vi "something test.vi"(8 "error in (no error)":errorcluster, 11 "Dummy In":refnum<class "Dummy.lvclass">) -> (0 "error out":errorcluster, 3 "Dummy Out":refnum<class "Dummy.lvclass">)   [LabVIEW 2020, in "Dummy.lvclass"]
uses:
  Dummy.lvclass
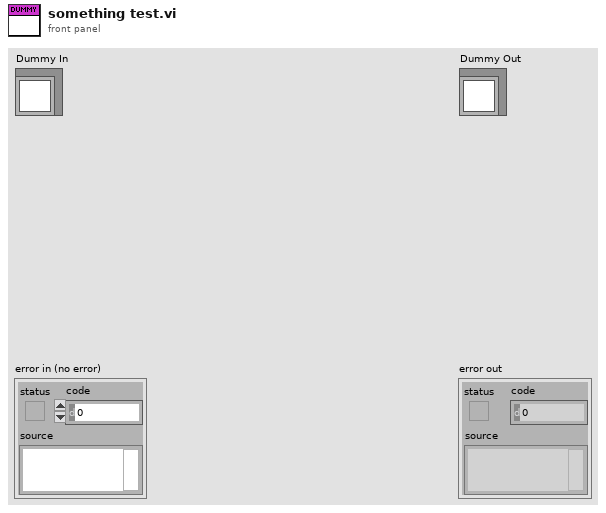
[diagram p1: front panel]
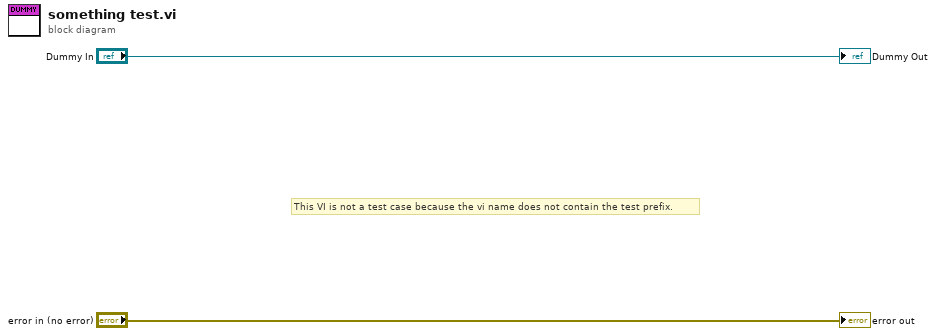
[diagram p0: block diagram]
diagram:
  # "This VI is not a test case because the vi name does not contain the test prefix."
  "error out" <- "error in (no error)"
  "Dummy Out" <- "Dummy In"
